vi "test Scaled and Unscaled.vi"(8 "error in (no error)":errorcluster, 11 "TestCase in":refnum<class "BNR.lvclass">) -> (0 "error out":errorcluster, 3 "TestCase out":refnum<class "BNR.lvclass">)   [LabVIEW 2027, in "BNR.lvclass"]
uses:
  BNR.lvclass
  b11c4b32-9ecc-4b3b-ab7a-55f1a6bc8d60.vi
  320dac47-5767-4d51-a5f7-ffdfdbb5a3b6.vi
  af2f1ac9-3d0e-4c86-9aa2-36521b937b88.vi
  e59510d1-05e5-469f-bc9b-27f0b4e077a0.vi
  320dac47-5767-4d51-a5f7-ffdfdbb5a3b6.vi/9377bb8f-44b5-4a8f-87f1-966fd5a9edcc.vi
  320dac47-5767-4d51-a5f7-ffdfdbb5a3b6.vi/e95d9d1f-307c-44d6-9f26-c3f519a4990d.vi
  320dac47-5767-4d51-a5f7-ffdfdbb5a3b6.vi/0c23f515-4369-4514-bc3d-4444e6b437b2.vi
  af2f1ac9-3d0e-4c86-9aa2-36521b937b88.vi/9377bb8f-44b5-4a8f-87f1-966fd5a9edcc.vi
  af2f1ac9-3d0e-4c86-9aa2-36521b937b88.vi/e95d9d1f-307c-44d6-9f26-c3f519a4990d.vi
  af2f1ac9-3d0e-4c86-9aa2-36521b937b88.vi/0c23f515-4369-4514-bc3d-4444e6b437b2.vi
  e59510d1-05e5-469f-bc9b-27f0b4e077a0.vi/16a2565b-3c16-407b-a626-9da2a3da432e.vi
  C:/Program Files/National Instruments/LabVIEW 2027/vi.lib/addons/_JKI Toolkits/VI Tester/TestCase.llb/TestCase.lvclass
  <vilib>/addons/_JKI Toolkits/VI Tester/TestCase.llb/TestCase.lvclass
panel:
  out "BCD encoded value":bool[](array[boolean])
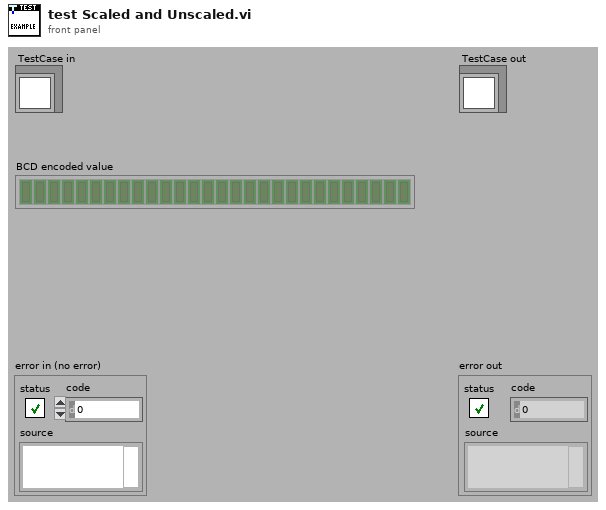
[diagram p1: front panel]
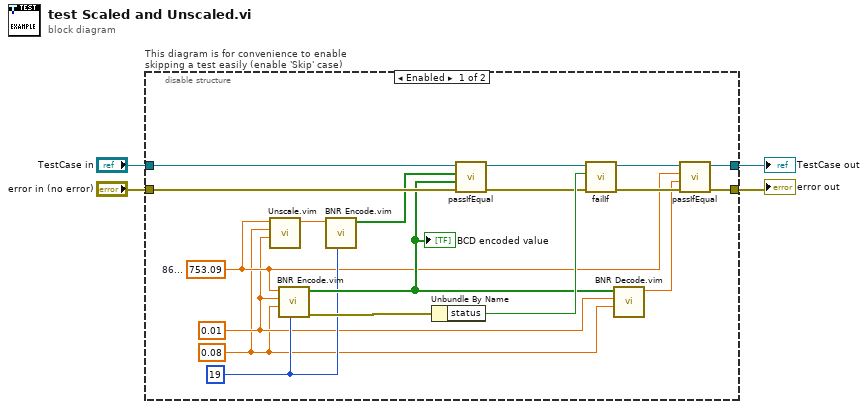
[diagram p0: block diagram]
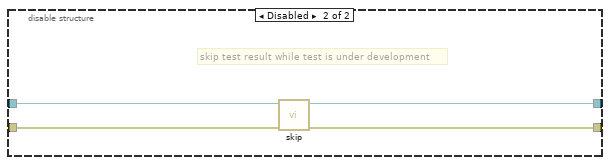
[diagram p2: hidden frame]
diagram:
  n1 = disable-structure "This diagram is for convenience to enable skipping a test easily (enable 'Skip' case)" shown="Enabled" {
    disable-tunnel: "TestCase in" -> [w22 w26]
    disable-tunnel: [w14 w24] -> w2
    disable-tunnel: [w15 w25] -> w3
    disable-tunnel: "error in (no error)" -> [w21 w23]
    frame Enabled {
      w6 = 0.08 ("scale multiplier")
      w7 = 0.01 ("scale multiplier")
      w10 = 19 ("data size (bits)")
      w8 = 753.09  # 86...
      n2 = call "Unscale.vim"("scale multiplier"=w7, "scale offset"=w6, "value"=w8) -> ("unscaled value"=w5:dbl)  [unwired: 8 in]
      n3 = call "BNR Encode.vim"("data size (bits)"=w10, "scale offset"=w6, "scale multiplier"=w7, "value"=w8) -> ("error out"=w11:errorcluster, "BNR encoded value"=w12:bool[])  [unwired: 6 in]
      "BCD encoded value" <- w12
      n4 = call "BNR Encode.vim"("data size (bits)"=w10, "value"=w5) -> ("BNR encoded value"=w9:bool[])  [unwired: 8 in, 1 out]
      n5 = Unbundle By Name(w11) -> ("status"=w20:bool)
      n6 = call-dynamic "passIfEqual.vi"("error in (no error)"=w21, "y"=w12, "x"=w9, "TestCase in"=w22) -> ("error out"=w18:errorcluster, "TestCase out"=w19:refnum<class "BNR.lvclass">)  [unwired: 6 in]
      n7 = call-dynamic "failIf.vi"("error in (no error)"=w18, "fail"=w20, "TestCase in"=w19) -> ("error out"=w16:errorcluster, "TestCase out"=w17:refnum<class "BNR.lvclass">)  [unwired: 7 in]
      n8 = call "BNR Decode.vim"("scale offset"=w6, "scale multiplier"=w7, "BNR encoded value"=w12) -> ("value"=w13:dbl)  [unwired: 8 in]
      n9 = call-dynamic "passIfEqual.vi"("error in (no error)"=w16, "y"=w13, "x"=w8, "TestCase in"=w17) -> ("error out"=w15:errorcluster, "TestCase out"=w14:refnum<class "BNR.lvclass">)  [unwired: 6 in]
    }
    frame Disabled {
      # "skip test result while test is under development"
      n10 = call <vilib>:"skip.vi"("error in (no error)"=w23, "TestCase in"=w26) -> ("error out"=w25:errorcluster, "TestCase out"=w24:refnum<class "BNR.lvclass">)  [unwired: 8 in]
    }
  }
  "error out" <- w3
  "TestCase out" <- w2
